vi "3.2.0 Kalman Covariance of Observation Noise Matrix R.vi"(1 "State Vector X":T1) -> (0 "Covariance of Observation Noise R":dbl[][](array[numeric]))   [LabVIEW 2010]
uses:
  4-High Neurons/4.2/4.2.0 Kalman State.ctl
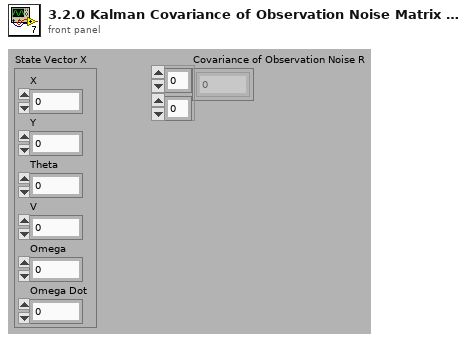
[diagram p1: front panel]
types:
  T1 = typedef "4.2.0 Kalman State.ctl" = cluster{"X":dbl, "Y":dbl, "Theta":dbl, "V":dbl, "Omega":dbl, "Omega Dot":dbl}
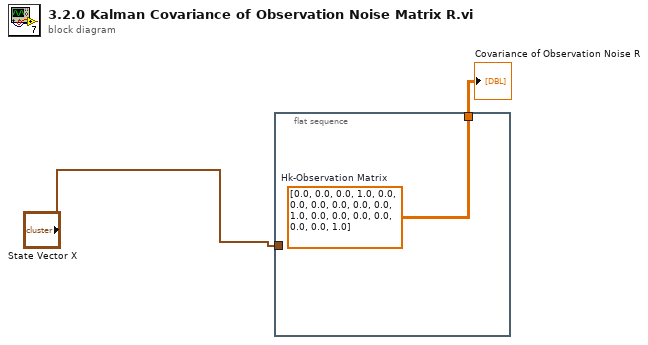
[diagram p0: block diagram]
diagram:
  n1 = flat-sequence {
    tunnel: "State Vector X" -> [_]
    tunnel: [w3] -> w2
    frame #0 {
      w3 = dbl[][] [[0.0, 0.0, 0.0, 1.0, 0.0, 0.0], [0.0, 0.0, 0.0, 0.0, 1.0, 0.0], [0.0, 0.0, 0.0, 0.0, 0.0, 1.0]]  # Hk-Observation Matrix
    }
  }
  "Covariance of Observation Noise R" <- w2
